vi "ProtekPvEmulator.vi"() -> ()   [LabVIEW 2016]
uses:
  <vilib>/Utility/file.llb/Read From Spreadsheet File (DBL).vi
panel:
  out "x+1":dbl
  out "abs(x)":dbl
  out "Döngü Time":u32
  out "Veriler Grafiği":T1(graph)
  out "Model_I":dbl
  out "Model_V":dbl
  out "e_I":dbl
  out "e_V":dbl
  out "NuData":i32
  out "GucK_R":dbl
  out "PgucK":dbl=60.0
  out "Vi Panel":dbl
  out "GucK_Com":bool
  out "GucK_W":dbl(knob) scale=0.0..60.0
  out "GucK_V":dbl(knob) scale=0.0..22.0
  in  "Port Sec":refnum<visa-resource-name>="COM1"
  out "GucK_I":dbl(knob) scale=0.0..3.7
  out "10_dk_ok":bool
  out "time":dbl
  out "i_Data":i32
  out "File patch":path
  out "Güç Grafiği":cluster{"PmaxM":dbl, "Pmaxe":dbl, "PgucK":dbl}(graph)
  in  "a":dbl=110.681443442253
  in  "Rs":dbl=25.0
  out "M_Pmax":dbl=60.29985558543294
  out "V - I Grafiği":cluster{"Vi":dbl, "Iint":dbl, dbl}(graph)={"Vi"=21.500000000000036, "Iint"=0.07178993987123095, 1.5434837072314678}
  in  "Rsh":dbl=110.681443442253
  in  "KV":dbl=-0.00863136
  in  "KI":dbl=0.0025624
  in  "ns":dbl=18.0
  out "e_Pmax":dbl=60.0
  in  "Voc":dbl=21.6
  in  "Isc":dbl=3.73
  in  "Vmp":dbl=17.3
  in  "Imp":dbl=3.47
  in  "G":dbl=1000.0
  in  "T":dbl=25.0
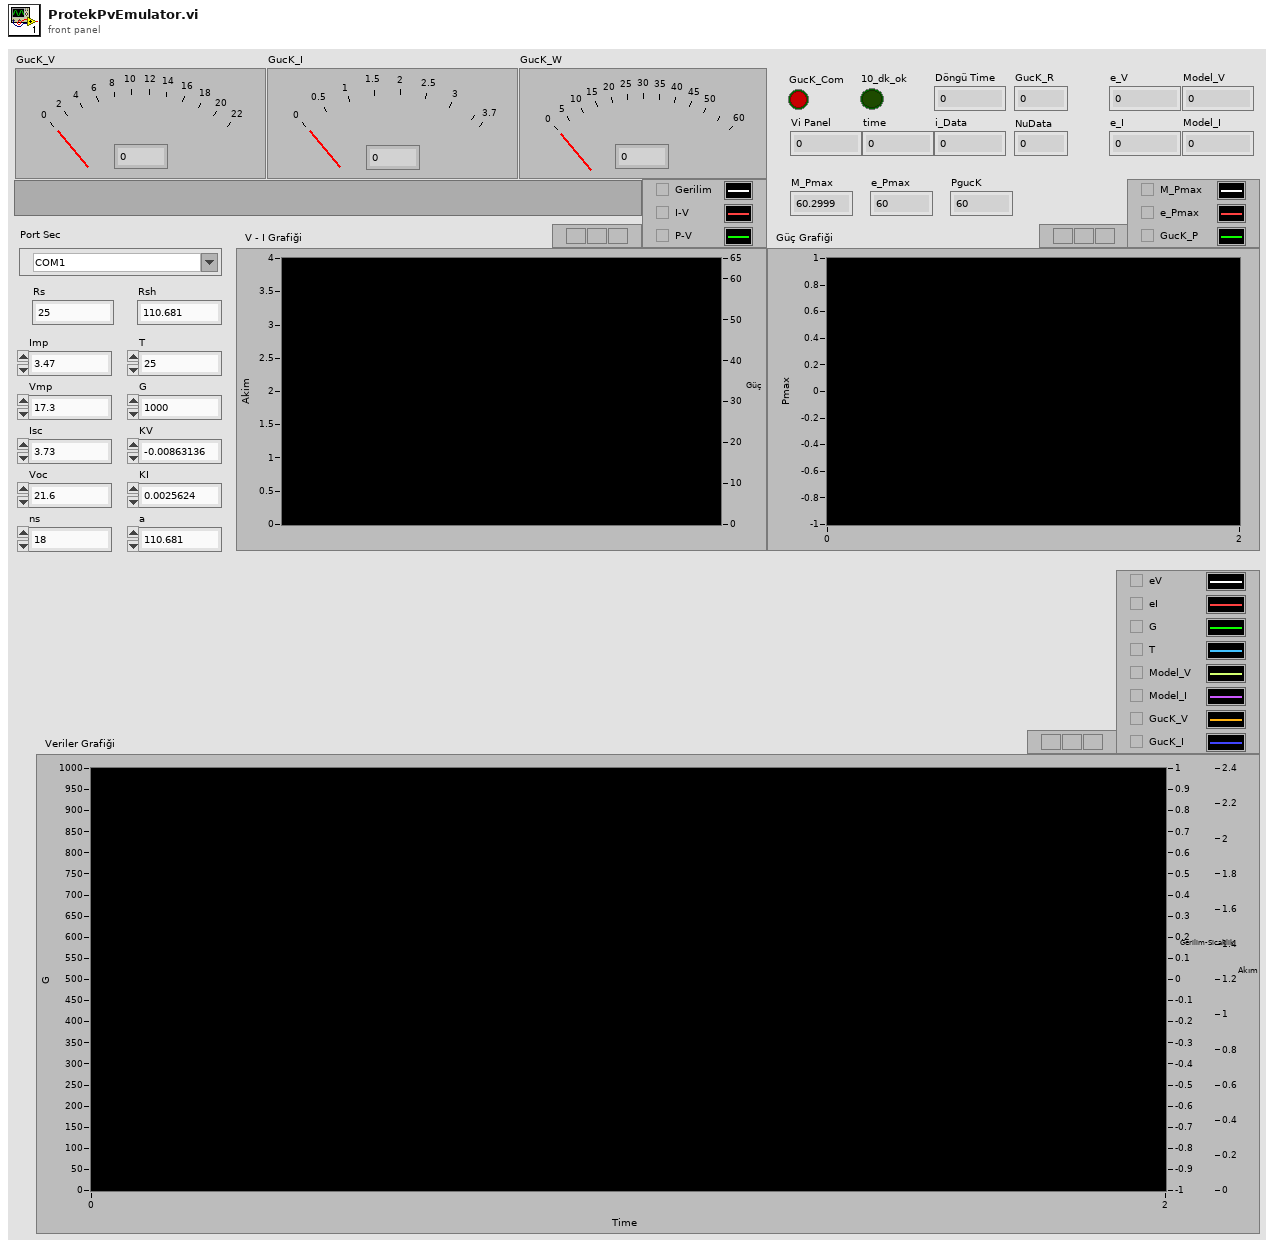
[diagram p1: front panel]
types:
  T1 = cluster{"e_V":dbl, "e_I":dbl, "G":dbl, "T":dbl, "Model_V":dbl, "Model_I":dbl, "GucK_V":dbl, "GucK_I":dbl}
  T2 = cluster{"e_V":dbl, "e_I":dbl, "G":dbl, "T":dbl, "Model_V":dbl, "Model_I":dbl, "GucK_V":dbl, "GucK_I":dbl}[]
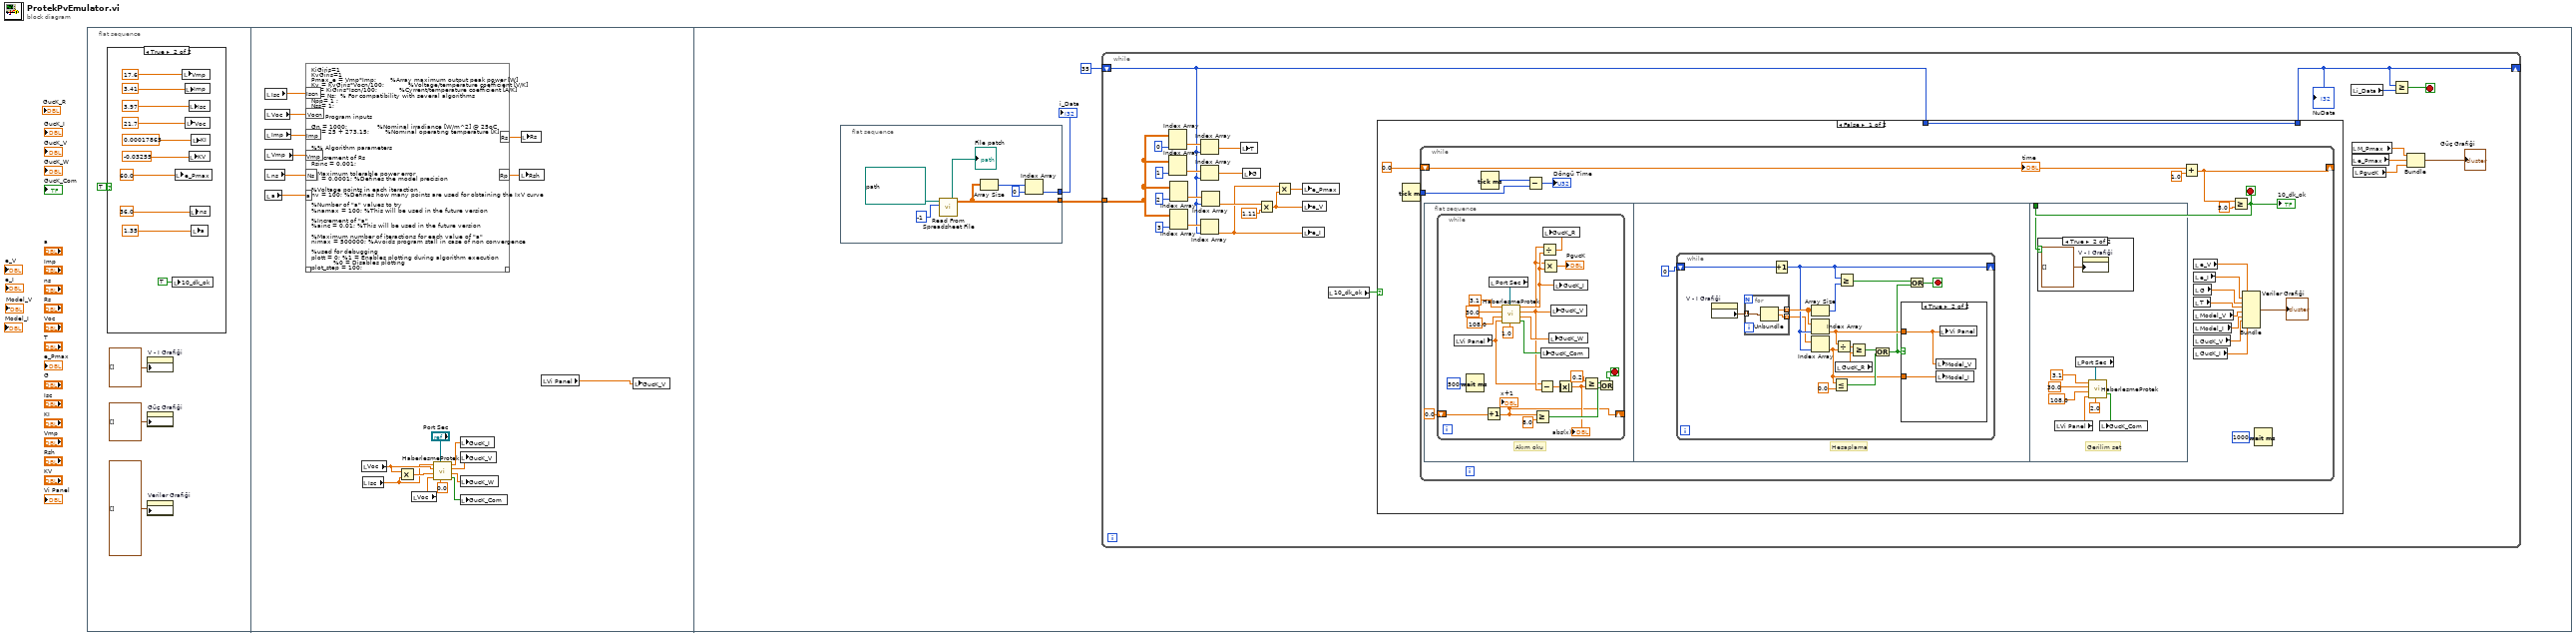
[diagram p0: block diagram]
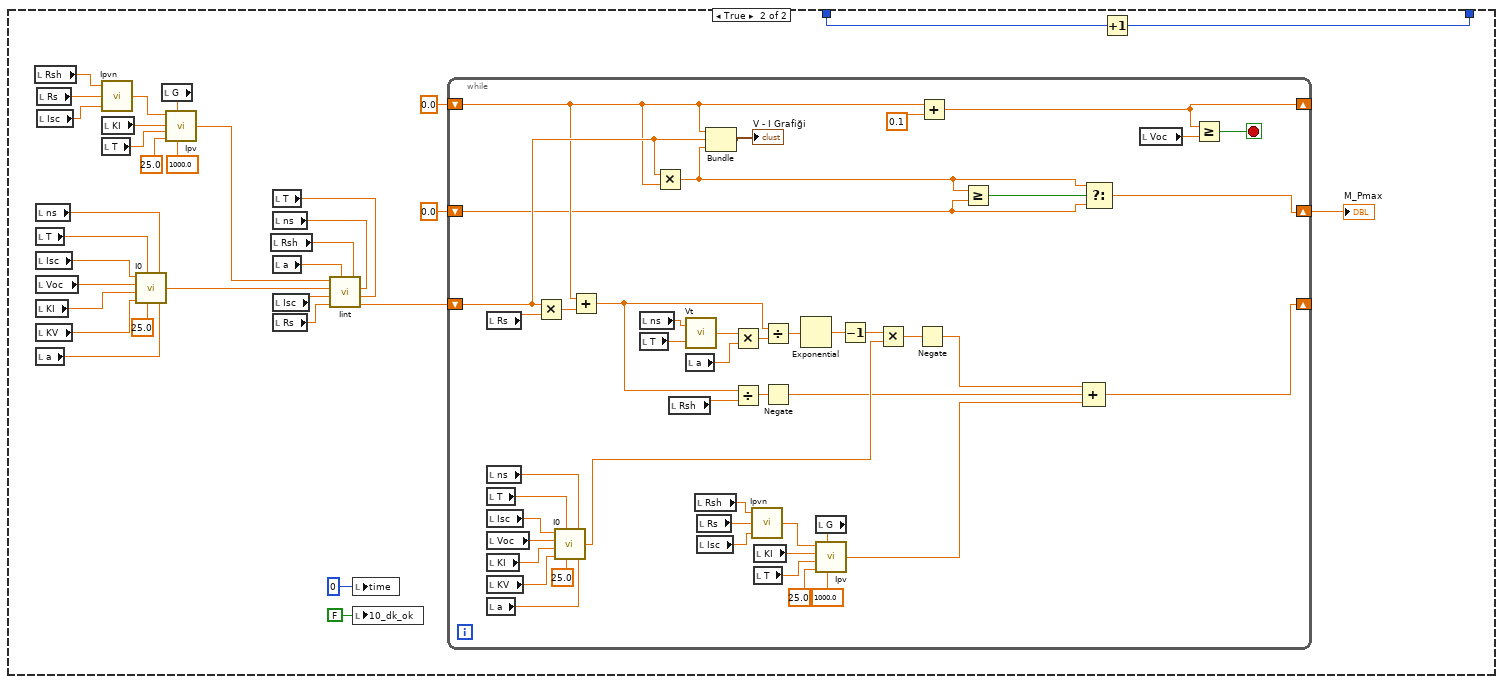
[diagram p5: hidden frame]
diagram:
  n1 = flat-sequence {
    frame #0 {
      n2 = case shown="True" TRUE {
        frame False {
        }
        frame True {
          n3 = local write "10_dk_ok"(TRUE ("10_dk_ok")) -> ()
          n4 = local write "e_Pmax"(60.0 ("Pmaxe")) -> ()
          n5 = local write "Vmp"(17.6 ("Vmp")) -> ()
          n6 = local write "Imp"(3.41 ("Imp")) -> ()
          n7 = local write "Voc"(21.7 ("Voc")) -> ()
          n8 = local write "Isc"(3.97 ("Isc")) -> ()
          n9 = local write "KV"(-0.03255 ("KV")) -> ()
          n10 = local write "ns"(36.0 ("ns")) -> ()
          n11 = local write "KI"(0.00017865 ("KI")) -> ()
          n12 = local write "a"(1.35 ("ns")) -> ()
        }
      }
      n13 = property on="V - I Grafiği" class="WFChart (strict)"("History Data"=cluster{"Vi":dbl, "Iint":dbl, dbl}[] []) -> ()  [unwired: 2 in, 2 out]
      n14 = property on="Güç Grafiği" class="WFChart (strict)"("History Data"=cluster{"PmaxM":dbl, "Pmaxe":dbl, "PgucK":dbl}[] []) -> ()  [unwired: 2 in, 2 out]
      n15 = property on="Veriler Grafiği" class="WFChart (strict)"("History Data"=T2 []) -> ()  [unwired: 2 in, 2 out]
    }
    frame #1 {
      n16 = local read "Isc"() -> (w29:dbl)
      n17 = local read "Voc"() -> (w26:dbl)
      n18 = local read "Imp"() -> (w30:dbl)
      n19 = local read "Vmp"() -> (w31:dbl)
      n20 = local read "ns"() -> (w32:dbl)
      n21 = local read "a"() -> (w33:dbl)
      n22 = script code="KiGiris=1\nKvGiris=1\nPmax_e = Vmp*Imp;       %Array maximum output peak power [W] \nKv = KvGiris*Vocn/100;            %Voltage/temperature coefficient [V/K] \nKi = KiGiris*Iscn/100;           %Cyrrent/temperature coefficient [A/K] \nns = Ns;  % For compatibility with several algorithms\nNpp= 1 ;\nNss= 1;\n \n%% Program inputs\n\nGn = 1000;               %Nominal irradiance [W/m^2] @ 25oC\nTn = 25 + 273.15;        %Nominal operating temperature [K]\n\n\n%% Algorithm parameters\n\n%Increment of Rs\nRsinc = 0.001;\n\n%Maximum tolerable power error\ntol = 0.0001; %Defines the model precision\n\n%Voltage points in each iteraction\nnv = 100; %Defines how many points are used for obtaining the IxV curve\n\n%Number of \"a\" values to try\n%namax = 100; %This will be used in the future version \n\n%Increment of \"a\"\n%ainc = 0.01; %This will be used in the future version \n\n%Maximum number of iteractions for each value of \"a\"\nnimax = 500000; %Avoids program stall in case of non convergence\n\n%used for debugging\nplott = 0; %1 = Enables plotting during algorithm execution\n           %0 = Disables plotting\nplot_step = 100;\n\n \n\n%% Adjusting algorithm\n\n% Reference values of Rs and Rp   \nRs_max = (Vocn - Vmp)/ Imp;\nRp_min = Vmp/(Iscn-Imp) - Rs_max;\n\n% Initial guesses of Rp and Rs\nRs = 0;\nRp = Rp_min;\n\n% The model is adjusted at the nominal condition\nT = Tn;\nG = Gn; \n\nk = 1.3806503e-23;   %Boltzmann [J/K]\nq = 1.60217646e-19;  %Electron charge [C]\n\nVtn = k * Tn / q;           %Thermal junction voltage (nominal) \nVt  = k * T  / q;           %Thermal junction voltage (current temperature)\n\n\nperror = Inf; %dummy value\n\n\n% Iterative process for Rs and Rp until Pmax,model = Pmax,experimental\n\nni = 0;\n\nwhile (perror>tol) && (Rp > 0) && (ni < nimax)\n\nni = ni + 1; \n    \n%  Temperature and irradiation effect on the current\ndT = T-Tn;\nIpvn = (Rs+Rp)/Rp * Iscn;         % Nominal light-generated current\nIpv = (Ipvn + Ki*dT) *G/Gn;       % Actual light-generated current \nIsc = (Iscn + Ki*dT) *G/Gn;       % Actual short-circuit current\n\nIo = (Ipv - Vocn/Rp)/(exp(Vocn/Vt/a/Ns)-1); %% NEW %% UPDATED ON JUNE/2010 %%\n\n% Increments Rs \nRs = Rs + Rsinc;  \n\nRp_ = Rp;\n\nRp = Vmp*(Vmp+Imp*Rs)/(Vmp*Ipv-Vmp*Io*exp((Vmp+Imp*Rs)/Vt/Ns/a)+Vmp*Io-Pmax_e);\n\n% Solving the I-V equation for several (V,I) pairs \n%clear V\n%clear I\n\nV = 0:Vocn/nv:Vocn;        % Voltage vector\nI = zeros(1,size(V,2));    % Current vector\n\nfor j = 1 : size(V,2) %Calculates for all voltage values \n    \n% Solves g = I - f(I,V) = 0 with Newton-Raphson\n  \ng(j) = Ipv-Io*(exp((V(j)+I(j)*Rs)/Vt/Ns/a)-1)-(V(j)+I(j)*Rs)/Rp-I(j);\n  \nwhile (abs(g(j)) > 0.001)\n      \ng(j) = Ipv-Io*(exp((V(j)+I(j)*Rs)/Vt/Ns/a)-1)-(V(j)+I(j)*Rs)/Rp-I(j);\nglin(j) = -Io*Rs/Vt/Ns/a*exp((V(j)+I(j)*Rs)/Vt/Ns/a)-Rs/Rp-1;\nI_(j) = I(j) - g(j)/glin(j);\nI(j) = I_(j);   \n  \nend  \n\nend % for j = 1 : size(V,2)\n\n%kapat\n%if (plott) \n    \n  %Plots the I-V and P-V curves\n\n  %Current x Voltage\n%  figure(1) \n% grid on\n%  hold on \n%  title('I-V curve - Adjusting Rs and Rp');\n%  xlabel('V [V]');\n%  ylabel('I [A]');\n%  xlim([0 Vocn]);\n%  ylim([0 Iscn]);\n \n  %Plots I x V curve\n%  plot(V,I,'LineWidth',2,'Color','k') \n \n  %Plots the \"remarkable points\" on the I x V curve\n%  plot([0 Vmp Vocn],[Iscn Imp 0],'o','LineWidth',2,'MarkerSize',5,'Color','k') \n\n  %Power x Voltage\n%  figure(2)  \n%  grid on\n%  hold on  \n%  title('P-V curve - Adjusting peak power');\n%  xlabel('V [V]');\n%  ylabel('P [W]');\n%  xlim([0 Vocn])\n%  ylim([0 Vmp*Imp]);\n    \n%end % if(plott)\n\n  % Calculates power using the I-V equation\n  P = (Ipv-Io*(exp((V+I.*Rs)/Vt/Ns/a)-1)-(V+I.*Rs)/Rp).*V;\n  \n  Pmax_m = max(P);\n  \n  perror = (Pmax_m-Pmax_e);\n\n%kapat  \n%if (plott) \n    \n  %Plots P x V curve\n%  plot(V,P,'LineWidth',2,'Color','k')\n  \n  %Plots the \"remarkable points\" on the power curve\n%  plot([0 Vmp Vocn],[0 Vmp*Imp 0],'o','LineWidth',2,'MarkerSize',5,'Color','k')\n  \n%end % if (plott)\n     \nend % while (error>tol) \n\nif (Rp<0) Rp = Rp_ \nend\n\nIon = Io; %\n\n\n%% Outputs\n \n % I-V curve\n% figure(3) \n% grid on\n% hold on \n% title('Adjusted I-V curve');\n% xlabel('V [V]');\n% ylabel('I [A]');\n% xlim([0 max(V)*1.1]);\n% ylim([0 max(I)*1.1]);\n \n% plot(V,I,'LineWidth',2,'Color','k') %\n% plot([0 Vmp Vocn ],[Iscn Imp 0 ],'o','LineWidth',2,'MarkerSize',5,'Color','k') \n \n % P-V curve\n\n% figure(4) \n% grid on\n% hold on \n% title('Adjusted P-V curve');\n% xlabel('V [V]');\n% ylabel('P [W]');\n% xlim([0 Vocn*1.1]);\n% ylim([0 Vmp*Imp*1.1]);\n  \n% plot(V,P,'LineWidth',2,'Color','k') %\n% plot([0 Vmp Vocn ],[0 Pmax_e 0 ],'o','LineWidth',2,'MarkerSize',5,'Color','k') \n   \n\n%disp(sprintf('Model info:\\n'));\n%disp(sprintf(' Rp_min = %f',Rp_min));\n%disp(sprintf('     Rp = %f',Rp));\n%disp(sprintf(' Rs_max = %f',Rs_max));\n%disp(sprintf('     Rs = %f',Rs));\n%disp(sprintf('      a = %f',a));\n%disp(sprintf('      T = %f',T-273.15));\n%disp(sprintf('      G = %f',G));\n%disp(sprintf(' Pmax,m = %f  (model)',Pmax_m));\n%disp(sprintf(' Pmax,e = %f  (experimental)',Pmax_e));\n%disp(sprintf('    tol = %f',tol));\n%disp(sprintf('P_error = %f',perror));\n%disp(sprintf('    Ipv = %f',Ipv));\n%disp(sprintf('    Isc = %f',Isc));\n%disp(sprintf('    Ion = %g',Ion));\n%disp(sprintf('    Ki = %g',Ki));\n%disp(sprintf('    Kv = %g',Kv));\n%disp(sprintf('\\n\\n'));\n\n\n%%% This feature is not available yet.\n%disp('Copy and paste this line of code in your simulation model:');\n%disp(sprintf('pvdata[14]={%f,%f,%f,%f,%f,%f,%f,%f,%f,%f,%f,%f,%f,%f};',Iscn,Vocn,Imp,Vmp,Kv,Ki,Ns,Gn,Tn,Rp,Rs,a,Ipvn,Ion));"("Iscn"=w29, "Vocn"=w26, "Imp"=w30, "Vmp"=w31, "Ns"=w32, "a"=w33) -> ("Rs"=w28:dbl, "Rp"=w27:dbl)  [unwired: 1 in, 1 out]
      n23 = local read "Voc"() -> (w18:dbl)
      n24 = local read "Isc"() -> (w17:dbl)
      n25 = Multiply(x=w18, y=w17) -> (x*y=w19:dbl)
      n26 = local read "Voc"() -> (w20:dbl)
      n27 = call "HaberlesmeProtek.vi"("Proses"=0.0, "VISA resource name"="Port Sec", "Voltaj set"=w20, "Max.Guc Set"=w19, "Max.Voltaj Set"=w18, "Max.Akım Set"=w17) -> ("checked data"=w25:bool, "Guc"=w24:dbl, "Voltaj"=w23:dbl, "Akım"=w22:dbl)  [unwired: 2 in]
      n28 = local write "GucK_I"(w22) -> ()
      n29 = local write "GucK_V"(w23) -> ()
      n30 = local write "GucK_W"(w24) -> ()
      n31 = local write "GucK_Com"(w25) -> ()
      n32 = local write "Rsh"(w27) -> ()
      n33 = local write "Rs"(w28) -> ()
      n34 = local read "Vi Panel"() -> (w15:dbl)
      n35 = local write "GucK_V"(w15) -> ()
    }
    frame #2 {
      n36 = flat-sequence {
        tunnel: [w40] -> w34
        tunnel: [w37] -> w35
        frame #0 {
          n37 = call-poly <vilib>:"Read From Spreadsheet File.vi"("number of rows (all:-1)"=-1, "file path (dialog if empty)"=path "D:/YüksekLisans/Tez/uygula/güneş paneli verileri/Tümü/Düzenlenen Veriler/Panel_6/P6Agustos30.xls") -> ("all rows"=w37:dbl[][], "new file path (Not A Path if cancelled)"=→"File patch":path)  [unwired: 2 in, 6 out]
          n38 = Array Size(array=w37) -> (size(s)=w41:i32[])
          n39 = Index Array(array=w41, index=0 ("index 2")) -> (element=w40:i32)
        }
      }
      n40 = while {
        shift-right: [w52] -> _
        shift-left: 35 -> [w51]
        tunnel: w35 -> [w56]
        stop <- w50 stop-if-true
        n41 = Index Array(array=w56, index (col)=0 ("disabled index (col)")) -> (element=w60:dbl[])  [unwired: 1 in]
        n42 = Index Array(array=w56, index (col)=1 ("disabled index (col)")) -> (element=w57:dbl[])  [unwired: 1 in]
        n43 = Index Array(array=w56, index (col)=2 ("disabled index (col)")) -> (element=w58:dbl[])  [unwired: 1 in]
        n44 = Index Array(array=w56, index (col)=3 ("disabled index (col)")) -> (element=w59:dbl[])  [unwired: 1 in]
        n45 = Index Array(array=w60, index=w51) -> (element=w54:dbl)
        n46 = Index Array(array=w57, index=w51) -> (element=w55:dbl)
        n47 = Index Array(array=w59, index=w51) -> (element=w44:dbl)
        n48 = Index Array(array=w58, index=w51) -> (element=w46:dbl)
        n49 = local write "T"(w54) -> ()
        n50 = local write "G"(w55) -> ()
        n51 = Multiply(x=w46, y=1.11) -> (x*y=w45:dbl)
        n52 = Multiply(x=w44, y=w45) -> (x*y=w47:dbl)
        n53 = local write "e_Pmax"(w47) -> ()
        n54 = local write "e_V"(w45) -> ()
        n55 = local write "e_I"(w44) -> ()
        n56 = local read "10_dk_ok"() -> (w53:bool)
        n57 = case shown="False" w53 {
          tunnel: [w70 w176] -> w52
          tunnel: w51 -> [w70 w175]
          frame False {
            n58 = Tick Count (ms)() -> (millisecond timer value=w69:u32)
            n59 = while {
              shift-right: [w72] -> _
              shift-left: 0.0 -> [w73]
              tunnel: w69 -> [w76]
              stop <- w87 stop-if-true
              n60 = flat-sequence {
                tunnel: w87 -> [w138]
                frame #0 {
                  # "Akım oku"
                  n61 = while {
                    shift-right: [w94] -> _
                    shift-left: 0.0 -> [w100]
                    stop <- w99 stop-if-true
                    n62 = local read "Vi Panel"() -> (w91:dbl)
                    n63 = Wait (ms)(milliseconds to wait=u32 500) -> ()  [unwired: 1 out]
                    n64 = Increment(x=w100) -> (x+1=w94:dbl)
                    "x+1" <- w94
                    n65 = local read "Port Sec"() -> (w103:refnum<visa-resource-name>)
                    n66 = call "HaberlesmeProtek.vi"("Proses"=1.0, "VISA resource name"=w103, "Voltaj set"=w91, "Max.Guc Set"=108.0, "Max.Voltaj Set"=30.0, "Max.Akım Set"=3.1) -> ("checked data"=w112:bool, "Guc"=w111:dbl, "Voltaj"=w92:dbl, "Akım"=w105:dbl)  [unwired: 2 in]
                    n67 = Greater Or Equal?(x=w94, y=8.0 ("x")) -> (x >= y?=w97:bool)
                    n68 = Subtract(x=w91, y=w92) -> (x-y=w102:dbl)
                    n69 = Divide(x=w92, y=w105) -> (x/y=w104:dbl)
                    n70 = local write "GucK_Com"(w112) -> ()
                    n71 = Multiply(x=w92, y=w105) -> (x*y=→"PgucK":dbl)
                    n72 = local write "GucK_R"(w104) -> ()
                    n73 = local write "GucK_W"(w111) -> ()
                    n74 = local write "GucK_V"(w92) -> ()
                    n75 = local write "GucK_I"(w105) -> ()
                    n76 = Absolute Value(x=w102) -> (abs(x)=w95:dbl)
                    "abs(x)" <- w95
                    n77 = Greater Or Equal?(x=0.2, y=w95) -> (x >= y?=w98:bool)
                    n78 = Or(x=w98, y=w97) -> (x .or. y?=w99:bool)
                  }
                }
                frame #1 {
                  # "Hesaplama"
                  n79 = while {
                    shift-right: [w124] -> _
                    shift-left: 0 -> [w127]
                    stop <- w120 stop-if-true
                    n80 = property on="V - I Grafiği" class="WFChart (strict)"() -> ("History Data"=w129:cluster{"Vi":dbl, "Iint":dbl, dbl}[])  [unwired: 2 in, 2 out]
                    n81 = for {
                      tunnel: w129 -> [w134] mode=indexing
                      tunnel: [w133] -> w128 mode=indexing
                      tunnel: [w132] -> w121 mode=indexing
                      n82 = Unbundle(w134) -> ("Vi"=w133:dbl, "Iint"=w132:dbl)  [unwired: 1 out]
                    }
                    n83 = Increment(x=w127) -> (x+1=w124:i32)
                    n84 = Array Size(array=w128) -> (size(s)=w126:i32)
                    n85 = Index Array(array=w128, index=w124) -> (element=w122:dbl)
                    n86 = Index Array(array=w121, index=w124) -> (element=w114:dbl)
                    n87 = Less Or Equal?(x=w114, y=0.0) -> (x <= y?=w117:bool)
                    n88 = Divide(x=w122, y=w114) -> (x/y=w123:dbl)
                    n89 = local read "GucK_R"() -> (w119:dbl)
                    n90 = Greater Or Equal?(x=w124, y=w126) -> (x >= y?=w125:bool)
                    n91 = Greater Or Equal?(x=w123, y=w119) -> (x >= y?=w116:bool)
                    n92 = Or(x=w116, y=w117) -> (x .or. y?=w115:bool)
                    n93 = case shown="True" w115 {
                      tunnel: w122 -> [_ w131]
                      tunnel: w114 -> [_ w130]
                      frame False {
                      }
                      frame True {
                        n94 = local write "Model_V"(w131) -> ()
                        n95 = local write "Model_I"(w130) -> ()
                        n96 = local write "Vi Panel"(w131) -> ()
                      }
                    }
                    n97 = Or(x=w125, y=w115) -> (x .or. y?=w120:bool)
                  }
                }
                frame #2 {
                  # "Gerilim set"
                  n98 = case shown="True" w138 {
                    frame False {
                    }
                    frame True {
                      n99 = property on="V - I Grafiği" class="WFChart (strict)"("History Data"=cluster{"Vi":dbl, "Iint":dbl, dbl}[] []) -> ()  [unwired: 2 in, 2 out]
                    }
                  }
                  n100 = local read "Vi Panel"() -> (w135:dbl)
                  n101 = local read "Port Sec"() -> (w137:refnum<visa-resource-name>)
                  n102 = call "HaberlesmeProtek.vi"("Proses"=2.0, "VISA resource name"=w137, "Voltaj set"=w135, "Max.Guc Set"=108.0 ("Max.Voltaj Set"), "Max.Voltaj Set"=30.0, "Max.Akım Set"=3.1) -> ("checked data"=w142:bool)  [unwired: 2 in, 3 out]
                  n103 = local write "GucK_Com"(w142) -> ()
                }
              }
              n104 = Tick Count (ms)() -> (millisecond timer value=w75:u32)
              n105 = Subtract(x=w75, y=w76) -> (x-y=→"Döngü Time":u32)
              n106 = Add(x=w73, y=1.0) -> (x+y=w72:dbl)
              n107 = local read "e_V"() -> (w78:dbl)
              n108 = local read "e_I"() -> (w79:dbl)
              n109 = local read "G"() -> (w80:dbl)
              n110 = local read "T"() -> (w81:dbl)
              n111 = local read "Model_V"() -> (w82:dbl)
              n112 = local read "Model_I"() -> (w83:dbl)
              n113 = local read "GucK_V"() -> (w84:dbl)
              n114 = local read "GucK_I"() -> (w85:dbl)
              n115 = Greater Or Equal?(x=w72, y=5.0) -> (x >= y?=w87:bool)
              "10_dk_ok" <- w87
              n116 = Bundle("e_V"=w78, "e_I"=w79, "G"=w80, "T"=w81, "Model_V"=w82, "Model_I"=w83, "GucK_V"=w84, "GucK_I"=w85) -> (→"Veriler Grafiği":T1)  [unwired: 1 in]
              n117 = Wait (ms)(milliseconds to wait=u32 1000) -> ()  [unwired: 1 out]
              "time" <- w73
            }
          }
          frame True {
            n118 = local read "Rsh"() -> (w153:dbl)
            n119 = local read "ns"() -> (w165:dbl)
            n120 = local read "T"() -> (w166:dbl)
            n121 = local read "Isc"() -> (w167:dbl)
            n122 = local read "Voc"() -> (w168:dbl)
            n123 = local read "KI"() -> (w169:dbl)
            n124 = local read "KV"() -> (w170:dbl)
            n125 = local read "a"() -> (w149:dbl)
            n126 = local read "Rs"() -> (w147:dbl)
            n127 = local read "Isc"() -> (w164:dbl)
            n128 = call "Ipvn.vi"("Iscn"=w164, "Rs"=w147, "Rp"=w153) -> ("Ipvn"=w159:dbl)
            n129 = local read "KI"() -> (w162:dbl)
            n130 = local read "T"() -> (w163:dbl)
            n131 = call "I0.vi"("Iscn"=w167, "T"=w166, "Vocn"=w168, "KI"=w169, "Tn"=25.0, "KV"=w170, "ns"=w165, "a"=w149) -> ("I0"=w157:dbl)
            n132 = local read "G"() -> (w151:dbl)
            n133 = call "Ipv.vi"("Gn"=1000.0, "G"=w151, "Tn"=25.0, "T"=w163, "KI"=w162, "Ipvn"=w159) -> ("Ipv"=w158:dbl)
            n134 = local read "Rsh"() -> (w152:dbl)
            n135 = local read "T"() -> (w173:dbl)
            n136 = local read "ns"() -> (w172:dbl)
            n137 = local read "a"() -> (w148:dbl)
            n138 = local read "Isc"() -> (w156:dbl)
            n139 = local read "Rs"() -> (w150:dbl)
            n140 = call "Iint.vi"("T"=w173, "ns"=w172, "Rp"=w152, "a"=w148, "Rs"=w150, "Isc"=w156, "I0"=w157, "Ipv"=w158) -> ("Iint"=w174:dbl)
            n141 = local write "time"(u32 0 ("time")) -> ()
            n142 = local write "10_dk_ok"(FALSE ("10_dk_ok")) -> ()
            n143 = while {
              shift-right: [w178] -> _
              shift-left: 0.0 -> [w189]
              shift-right: [w199] -> _
              shift-left: w174 -> [w190]
              shift-right: [w187] -> w154
              shift-left: 0.0 -> [w186]
              stop <- w192 stop-if-true
              n144 = local read "Rs"() -> (w179:dbl)
              n145 = local read "ns"() -> (w217:dbl)
              n146 = local read "T"() -> (w216:dbl)
              n147 = local read "Isc"() -> (w215:dbl)
              n148 = local read "Voc"() -> (w214:dbl)
              n149 = local read "KI"() -> (w213:dbl)
              n150 = local read "KV"() -> (w212:dbl)
              n151 = local read "a"() -> (w180:dbl)
              n152 = Multiply(x=w190, y=w179) -> (x*y=w206:dbl)
              n153 = call "I0.vi"("Iscn"=w215, "T"=w216, "Vocn"=w214, "KI"=w213, "Tn"=25.0, "KV"=w212, "ns"=w217, "a"=w180) -> ("I0"=w201:dbl)
              n154 = Add(x=w189, y=w206) -> (x+y=w200:dbl)
              n155 = local read "ns"() -> (w208:dbl)
              n156 = local read "T"() -> (w209:dbl)
              n157 = Multiply(x=w190, y=w189) -> (x*y=w177:dbl)
              n158 = local read "Rsh"() -> (w185:dbl)
              n159 = call "Vt.vi"("T"=w209, "ns"=w208) -> ("Vt"=w207:dbl)
              n160 = local read "a"() -> (w181:dbl)
              n161 = local read "Rsh"() -> (w183:dbl)
              n162 = local read "Rs"() -> (w184:dbl)
              n163 = local read "Isc"() -> (w218:dbl)
              n164 = Bundle(w189, "Iint"=w190, w177) -> (→"V - I Grafiği":cluster{dbl, "Iint":dbl, dbl})  [unwired: 1 in]
              n165 = Multiply(x=w207, y=w181) -> (x*y=w205:dbl)
              n166 = Divide(x=w200, y=w185) -> (x/y=w194:dbl)
              n167 = call "Ipvn.vi"("Iscn"=w218, "Rs"=w184, "Rp"=w183) -> ("Ipvn"=w223:dbl)
              n168 = local read "KI"() -> (w220:dbl)
              n169 = local read "T"() -> (w219:dbl)
              n170 = Divide(x=w200, y=w205) -> (x/y=w204:dbl)
              n171 = Negate(x=w194) -> (-x=w195:dbl)
              n172 = Exponential(1:w204) -> (0:w203:dbl)
              n173 = local read "G"() -> (w182:dbl)
              n174 = call "Ipv.vi"("Gn"=1000.0, "G"=w182, "Tn"=25.0, "T"=w219, "KI"=w220, "Ipvn"=w223) -> ("Ipv"=w198:dbl)
              n175 = Decrement(x=w203) -> (x-1=w202:dbl)
              n176 = Multiply(x=w202, y=w201) -> (x*y=w197:dbl)
              n177 = Negate(x=w197) -> (-x=w196:dbl)
              n178 = Add(x=w189, y=0.1) -> (x+y=w178:dbl)
              n179 = Greater Or Equal?(x=w177, y=w186) -> (x >= y?=w188:bool)
              n180 = Compound Arithmetic op=ADD(w196, w195, w198) -> (w199:dbl)
              n181 = Select(t=w177, s=w188, f=w186) -> (s? t:f=w187:dbl)
              n182 = local read "Voc"() -> (w193:dbl)
              n183 = Greater Or Equal?(x=w178, y=w193) -> (x >= y?=w192:bool)
            }
            "M_Pmax" <- w154
            n184 = Increment(x=w175) -> (x+1=w176:i32)
          }
        }
        "NuData" <- w52
        n185 = local read "i_Data"() -> (w68:i32)
        n186 = local read "M_Pmax"() -> (w66:dbl)
        n187 = local read "e_Pmax"() -> (w65:dbl)
        n188 = local read "PgucK"() -> (w49:dbl)
        n189 = Greater Or Equal?(x=w52, y=w68) -> (x >= y?=w50:bool)
        n190 = Bundle("M_Pmax"=w66, "e_Pmax"=w65, "PgucK"=w49) -> (→"Güç Grafiği":cluster{"M_Pmax":dbl, "e_Pmax":dbl, "PgucK":dbl})  [unwired: 1 in]
      }
      "i_Data" <- w34
    }
  }
